vi "Raw Text to String.vi"(8 "Error In":errorcluster, 9 "Use Example Input":bool, 10 "Example Input":string, 11 "Relative Path to Input File":string) -> (0 "Error Out":errorcluster, 3 "String":string)   [LabVIEW 2019]
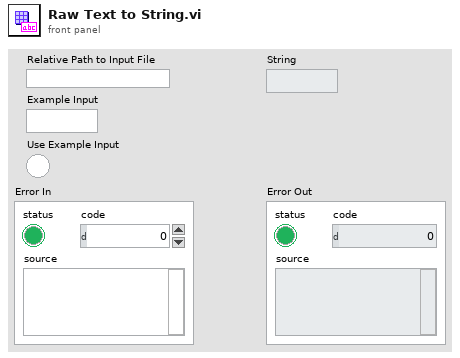
[diagram p1: front panel]
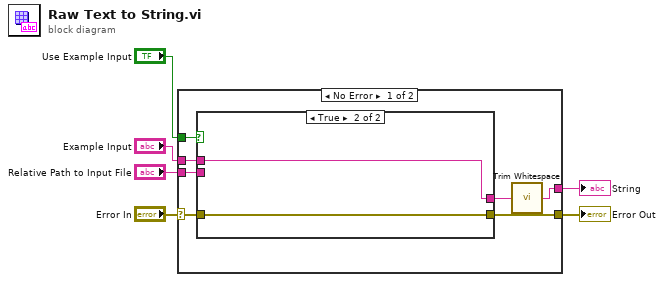
[diagram p0: block diagram]
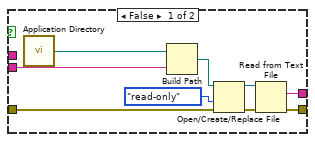
[diagram p2: hidden frame]
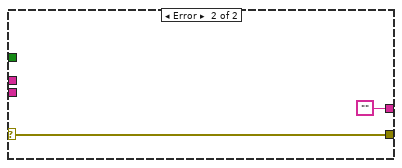
[diagram p3: hidden frame]
diagram:
  n1 = case shown="No Error" "Error In" {
    selector: "Error In" -> [w11 w26]
    tunnel: "Relative Path to Input File" -> [w13 _]
    tunnel: [w7 ""] -> w1
    tunnel: [w12 w26] -> w3
    tunnel: "Use Example Input" -> [w10 _]
    tunnel: "Example Input" -> [w9 _]
    frame No Error {
      n2 = case shown="True" w10 {
        tunnel: w13 -> [w21 _]
        tunnel: [w16 w24] -> w8
        tunnel: [w15 w23] -> w12
        tunnel: w11 -> [w14 w23]
        tunnel: w9 -> [_ w24]
        frame False {
          n3 = call <vilib>:"Application Directory.vi"() -> ("Application Directory"=w22:path)
          n4 = Build Path(base path=w22, name or relative path=w21) -> (appended path=w20:path)
          n5 = Open/Create/Replace File(file path (use dialog)=w20, error in=w14, access (0:read/write)=enum16{"read/write", "read-only", "write-only"}."read-only") -> (refnum out=w18:refnum<file>, error out=w17:errorcluster)  [unwired: 3 in, 1 out]
          n6 = Read from Text File(file (use dialog)=w18, error in=w17) -> (text=w16:string, error out=w15:errorcluster)  [unwired: 2 in, 2 out]
        }
        frame True {
        }
      }
      n7 = call <vilib>:"Trim Whitespace.vi"("string"=w8) -> ("trimmed string"=w7:string)  [unwired: 1 in]
    }
    frame Error {
    }
  }
  "Error Out" <- w3
  "String" <- w1
